vi "Test Digital Integrator.vi"() -> ()   [LabVIEW 2020]
panel:
  out "?":dbl[](array[numeric])=[0.00013280642653537187] format="%.4f"
  in  "Instrument Address":refnum<visa-resource-name>="GPIB0::4::INSTR"
  in  "stop":bool
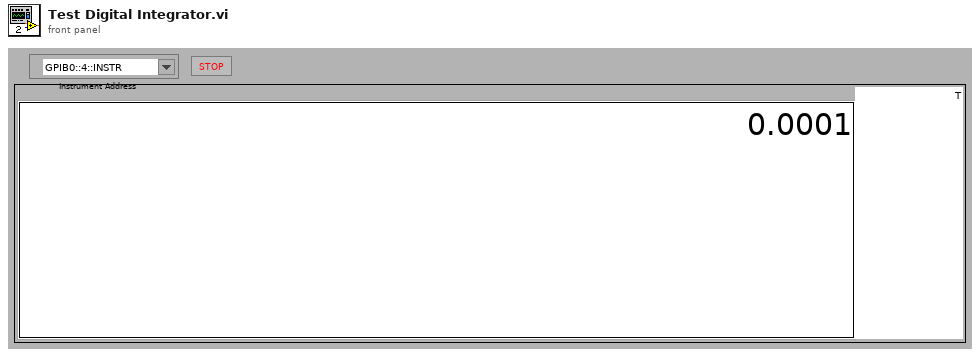
[diagram p1: front panel]
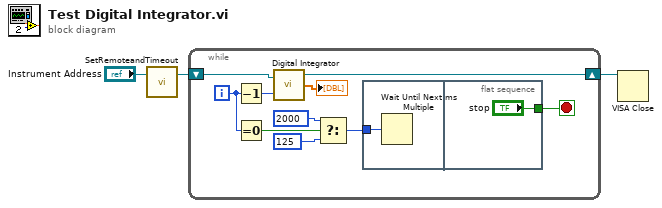
[diagram p0: block diagram]
diagram:
  n1 = call "SetRemoteandTimeout.vi"("VISA resource"="Instrument Address") -> ("dup VISA resource"=w2:refnum<visa-resource-name>)  [unwired: 1 in, 1 out]
  n2 = while {
    shift-right: [w4] -> w1
    shift-left: w2 -> [w5]
    i -> [w6]
    stop <- w11 stop-if-true
    n3 = Decrement(x=w6) -> (x-1=w13:i32)
    n4 = Equal To 0?(x=w6) -> (x = 0?=w10:bool)
    n5 = call "Digital Integrator.vi"("Instrument Address"=w5, "Index"=w13) -> ("dup VISA Session"=w4:refnum<visa-resource-name>, 3:→"?":dbl[])  [unwired: 1 out]
    n6 = Select(t=u32 2000 ("millisecond multiple"), s=w10, f=u32 125) -> (s? t:f=w9:u32)
    n7 = flat-sequence {
      tunnel: w9 -> [w14]
      tunnel: ["stop"] -> w11
      frame #0 {
        n8 = Wait Until Next ms Multiple(millisecond multiple=w14) -> ()  [unwired: 1 out]
      }
      frame #1 {
      }
    }
  }
  n9 = VISA Close(VISA resource name=w1) -> ()  [unwired: 1 in, 1 out]
